vi "aula2.vi"() -> ()   [LabVIEW 2024]
panel:
  in  "Numeric":dbl
  in  "stop 2":bool
  out "Qtd de Execução 2":dbl
  in  "° F 2":dbl(slide) scale=-40.0..212.0
  out "° C 2":dbl(slide) scale=0.0..100.0
  in  "Boolean":bool
  out "Qtd de Execução":dbl
  out "° C":dbl(slide) scale=0.0..100.0
  in  "° F":dbl(slide) scale=-40.0..212.0
  in  "stop":bool
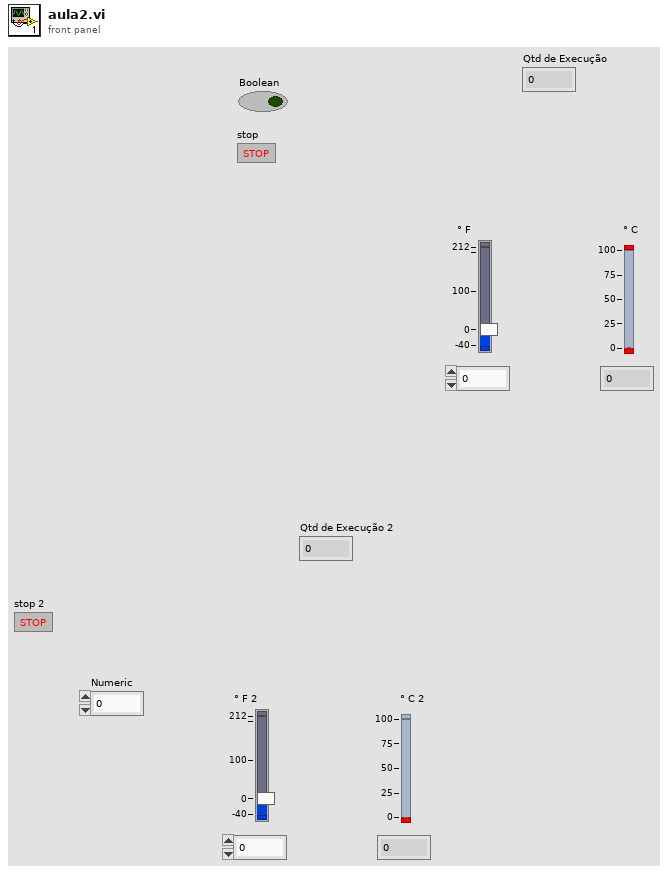
[diagram p1: front panel]
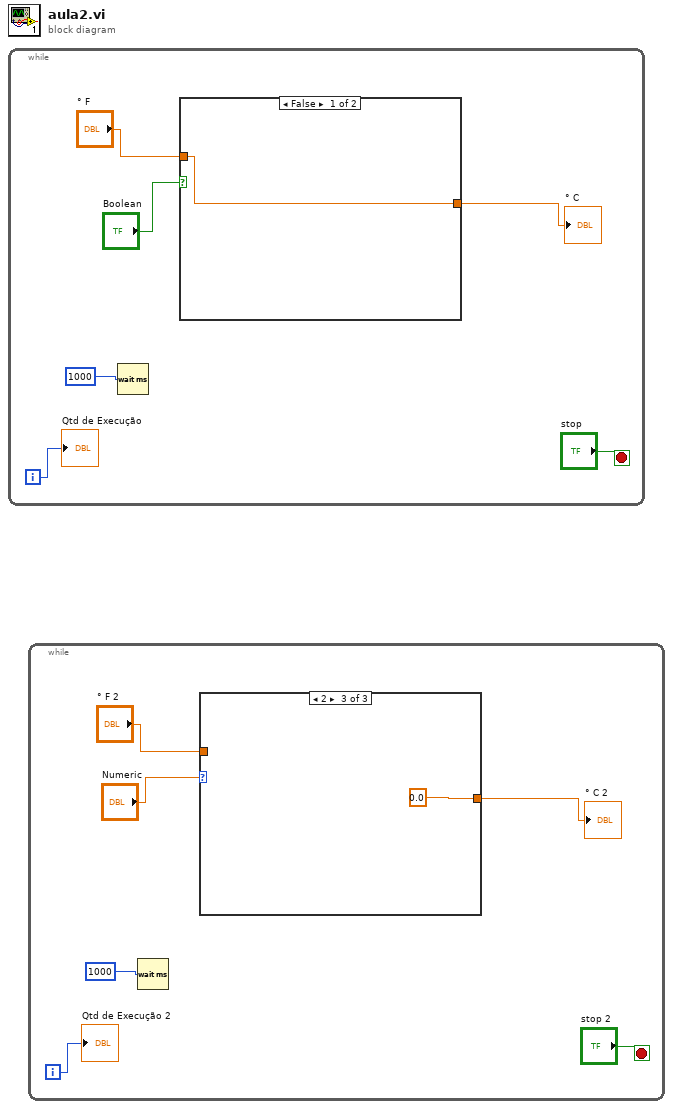
[diagram p0: block diagram]
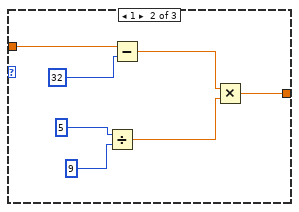
[diagram p3: hidden frame]
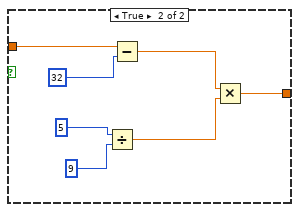
[diagram p4: hidden frame]
diagram:
  n1 = while {
    i -> [w4]
    stop <- "stop" stop-if-true
    n2 = Wait (ms)(milliseconds to wait=1000) -> ()  [unwired: 1 out]
    n3 = case shown="False" "Boolean" {
      tunnel: "° F" -> [w7 w9]
      tunnel: [w7 w8] -> w2
      frame False {
      }
      frame True {
        n4 = Divide(x=5, y=9) -> (x/y=w10:dbl)
        n5 = Subtract(x=w9, y=32) -> (x-y=w11:dbl)
        n6 = Multiply(x=w11, y=w10) -> (x*y=w8:dbl)
      }
    }
    "° C" <- w2
    "Qtd de Execução" <- w4
  }
  n7 = while {
    i -> [w18]
    stop <- "stop 2" stop-if-true
    n8 = Wait (ms)(milliseconds to wait=1000) -> ()  [unwired: 1 out]
    n9 = case shown="2" "Numeric" {
      tunnel: "° F 2" -> [w21 w23 _]
      tunnel: [w21 w22 0.0 ("° F 2")] -> w16
      frame 0, Default {
      }
      frame 1 {
        n10 = Divide(x=5, y=9) -> (x/y=w24:dbl)
        n11 = Subtract(x=w23, y=32) -> (x-y=w25:dbl)
        n12 = Multiply(x=w25, y=w24) -> (x*y=w22:dbl)
      }
      frame 2 {
      }
    }
    "° C 2" <- w16
    "Qtd de Execução 2" <- w18
  }
